vi "actionFrontEnd.vi"(6 "index":i32, 7 "editing":bool, 8 "error in (no error)":errorcluster, 9 "deviceDataBase":refnum<class "deviceDataBase.lvclass">, 10 "ScriptEventList":refnum<class "ScriptEventList.lvclass">, 11 "ActionEditor in":refnum<class "ActionEditor.lvclass">) -> (0 "error out":errorcluster, 1 "canceled":bool, 2 "ScriptEventList out":refnum<class "ScriptEventList.lvclass">, 3 "ActionEditor out":refnum<class "ActionEditor.lvclass">)   [LabVIEW 2009, in "Views.lvlib" / "ScriptEditor.lvlib" / "ActionEditor.lvclass"]
uses:
  ActionEditor.lvclass
  Tools/Scripting/ScriptingEvent/ScriptEventList/ScriptEventList.lvclass
  Tools/DatabaseHelpers/DbConnection/DeviceDataBase/deviceDataBase.lvclass
  ActionEditor.lvclass/ActionEditor.ctl
  Tools/Scripting/ScriptingEvent/ScriptEvent.lvclass
  Tools/DatabaseHelpers/Database Objects/ChannelArray/ChannelArray.lvclass
panel:
  in  "AfterEventBox":i32(listbox)
  in  "BeforeEventBox":i32[](listbox)
  in  "Stage":T1(ring)
  in  "Units":string
  in  "Delay All Events?":bool=TRUE
  in  "Comment":string
  in  "OK Button":bool
  in  "Cancel Button":bool
  in  "Channel Name":u16(ring) items=["", "Cooling_Detuning", "MOT coil", "analog2", "analog3", "analog4", "analog5", "analog6", "analog7", "analogB0", "analogB1", "analogB2", "analogB3", "analogB4", "analogB5", "analogB6", "analogB7", "Pixelfly_trigger", "Coil_Switch", "Cooling_Shutter", "Repump_Shutter", "SpinCoreDDS0_rf_trigger", "SpinCoreDDS1_rf_trigger", "CQTDDS0_rf_trigger", "Repump_AOM", "Cooling_AOM", "Imaging_Aom", "TiS", "cDDS_00", "cDDS_01", "ethernet0", "ethernet1", "ethernet2", "ethernet3"]
  in  "Action":T2(ring)
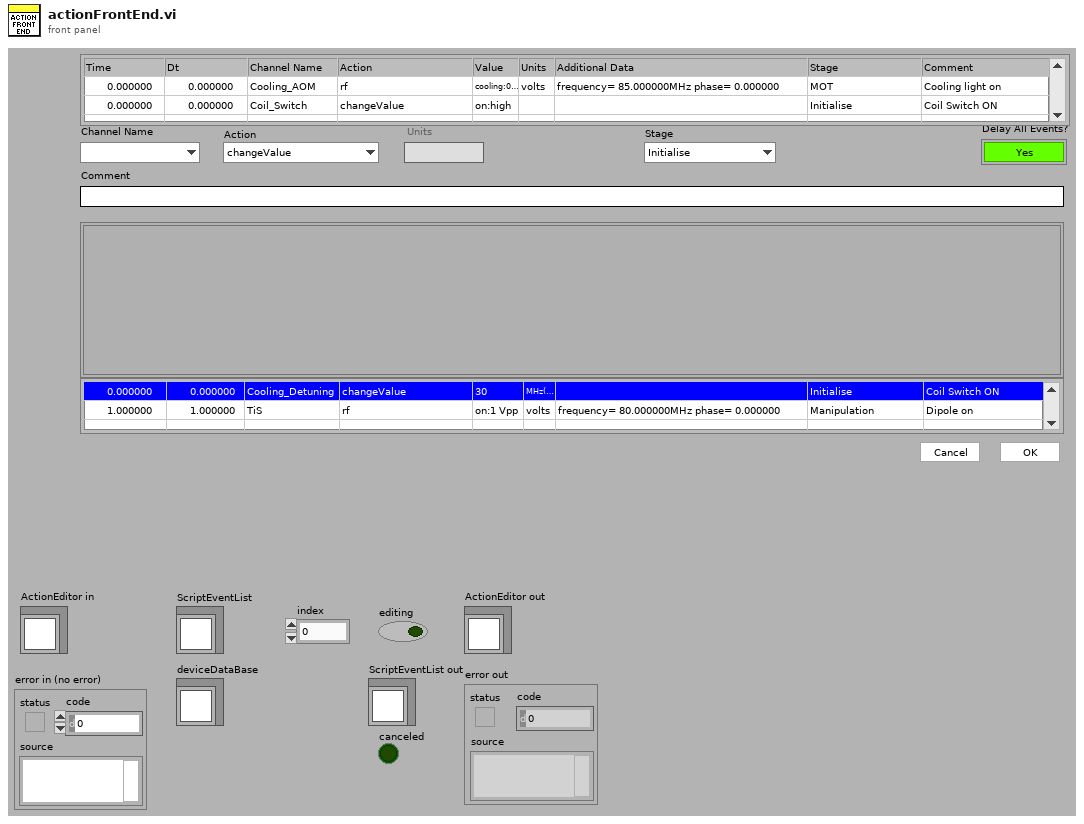
[diagram p1: front panel]
types:
  T1 = enum16{"Initialise", "MOT", "Molasses", "Optical Pumping", "Magnetic Trap", "RF Cooling", "Manipulation", "Switch Off", "Absorption Imaging", "Fluorscence Imaging", "Shut Down"}
  T2 = enum16{"changeValue", "pulse", "clock", "rampUp", "rampDown", "singleTone", "singleToneRamp", "playFile", "rf", "rfRamp"}
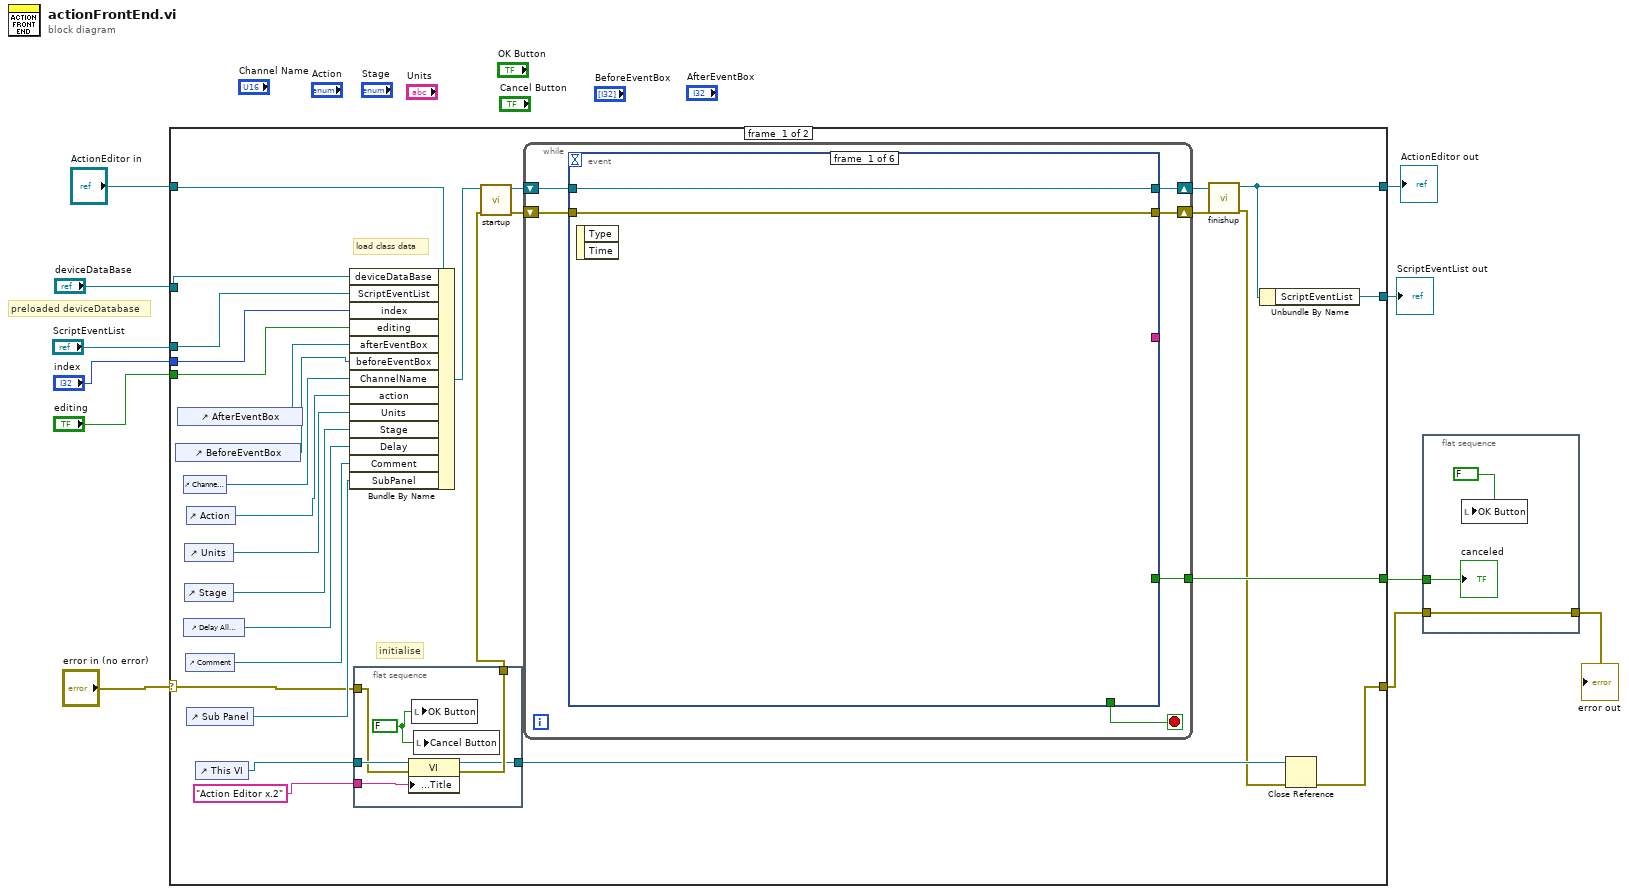
[diagram p0: block diagram]
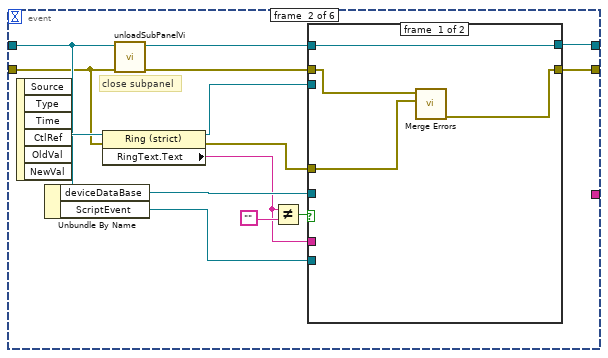
[diagram p2: hidden frame]
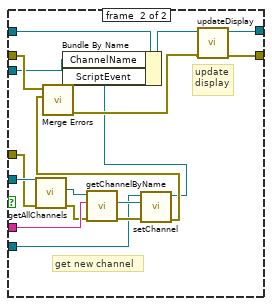
[diagram p3: hidden frame]
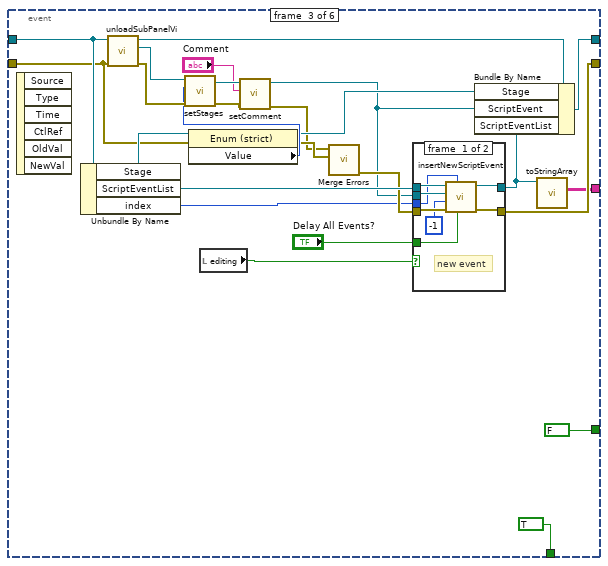
[diagram p4: hidden frame]
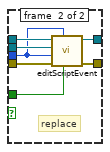
[diagram p5: hidden frame]
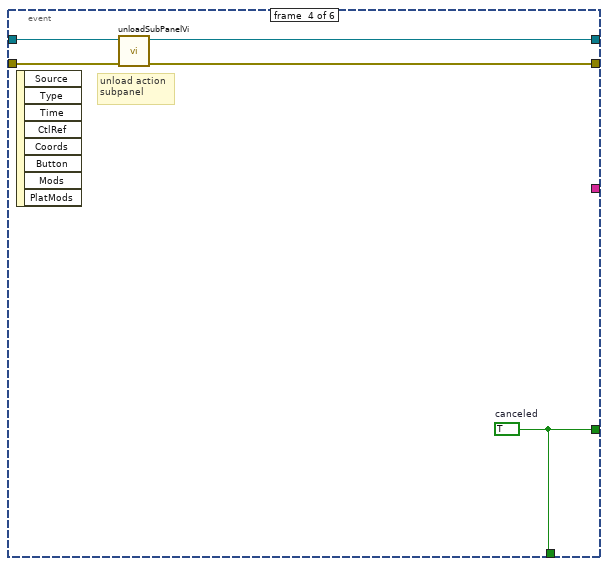
[diagram p6: hidden frame]
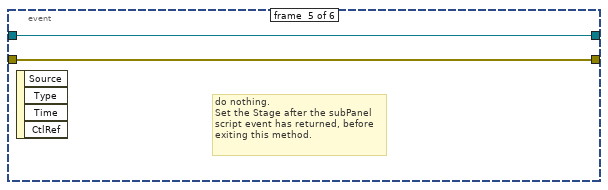
[diagram p7: hidden frame]
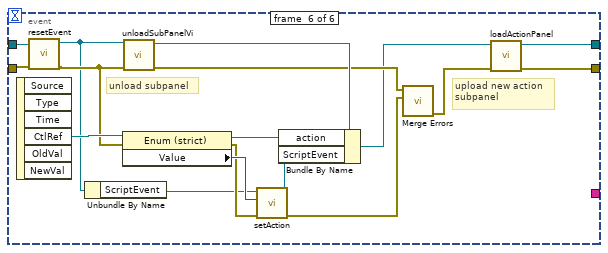
[diagram p8: hidden frame]
diagram:
  # "preloaded deviceDatabase"
  n1 = case shown="No Error" "error in (no error)" {
    selector: "error in (no error)" -> [w20 w155]
    tunnel: [w13 w155] -> w3
    tunnel: [w23 w154] -> w9
    tunnel: "ActionEditor in" -> [w36 w154]
    tunnel: "deviceDataBase" -> [w35 _]
    tunnel: "ScriptEventList" -> [w33 _]
    tunnel: "index" -> [w32 _]
    tunnel: [w24 _] -> w5
    tunnel: [w22 _] -> w4
    tunnel: "editing" -> [w18 _]
    frame #0 {
      # "initialise"
      # "load class data"
      n2 = control-ref of="BeforeEventBox"() -> (w21:refnum<vi>)
      n3 = control-ref of="AfterEventBox"() -> (w31:refnum<vi>)
      n4 = control-ref of="Channel Name"() -> (w30:refnum<vi>)
      n5 = control-ref of="Delay All Events?"() -> (w27:refnum<vi>)
      n6 = control-ref of="Units"() -> (w29:refnum<vi>)
      n7 = control-ref of="Stage"() -> (w28:refnum<vi>)
      n8 = control-ref of="Comment"() -> (w26:refnum<vi>)
      n9 = control-ref of="Action"() -> (w12:refnum<vi>)
      n10 = control-ref of="Sub Panel"() -> (w25:refnum<vi>)
      n11 = control-ref of="This VI"() -> (w17:refnum<vi>)
      n12 = Bundle By Name(cluster=w36, "deviceDataBase"=w35, "ScriptEventList"=w33, "index"=w32, "editing"=w18, "afterEventBox"=w31, "beforeEventBox"=w21, "ChannelName"=w30, "action"=w12, "Units"=w29, "Stage"=w28, "Delay"=w27, "Comment"=w26, "SubPanel"=w25) -> (w34:refnum<class "ActionEditor.lvclass">)
      n13 = flat-sequence {
        tunnel: w20 -> [w44]
        tunnel: [w43] -> w19
        tunnel: w17 -> [w45]
        tunnel: [w42] -> w15
        tunnel: "Action Editor x.2" -> [w41]
        frame #0 {
          w46 = FALSE
          n14 = property class="VI"(reference=w45, error in=w44, "Front Panel.Title"=w41) -> (reference out=w42:refnum<vi>, error out=w43:errorcluster)
          n15 = local write "OK Button"(w46) -> ()
          n16 = local write "Cancel Button"(w46) -> ()
        }
      }
      n17 = call "startup.vi"("error in (no error)"=w19, "ActionEditor in"=w34) -> ("error out"=w39:errorcluster, "ActionEditor out"=w40:refnum<class "ActionEditor.lvclass">)  [unwired: 8 in]
      n18 = while {
        shift-right: [w51] -> w37
        shift-left: w40 -> [w52]
        shift-right: [w49] -> w38
        shift-left: w39 -> [w50]
        tunnel: [w47] -> w24
        stop <- w48 stop-if-true
        n19 = event shown="[5] \"Action\": Value Change" {
          selector: _ -> [_ _ _ _ _ _]
          dyn-events: _ -> [_ _ _ _ _ _]
          timeout: _ -> [_ _ _ _ _ _]
          tunnel: [w54 w57 w100 w133 w136 w146] -> w51
          tunnel: w52 -> [w54 w67 w113 w131 w136 w140]
          tunnel: w50 -> [w53 w66 w109 w134 w135 w139]
          tunnel: [w53 w56 w102 w132 w135 w145] -> w49
          tunnel: [_ _ TRUE w130 _ _] -> w48
          tunnel: [_ _ FALSE w130 _ _] -> w47
          tunnel: [_ _ w90 _ _ _] -> _
          event #0 {
            n20 = event-data() -> ()  [unwired: 1 in, 2 out]
          }
          event #1 {
            # "close subpanel"
            n21 = event-data() -> ("CtlRef"=w68:refnum<vi>)  [unwired: 1 in, 5 out]
            n22 = Unbundle By Name(w67) -> ("deviceDataBase"=w62:refnum<class "deviceDataBase.lvclass">, "ScriptEvent"=w60:refnum<class "ScriptEvent.lvclass">)
            n23 = property class="Ring (strict)"(reference=w68, error in=w66) -> (reference out=w55:refnum<vi>, error out=w63:errorcluster, "RingText.Text"=w61:string)
            n24 = call "unloadSubPanelVi.vi"("error in (no error)"=w66, "ActionEditor in"=w67) -> ("error out"=w58:errorcluster, "ActionEditor out"=w59:refnum<class "ActionEditor.lvclass">)  [unwired: 6 in, 2 out]
            n25 = Not Equal?(x=w61, y="") -> (x != y?=w65:bool)
            n26 = case shown="True" w65 {
              tunnel: w63 -> [w70 w88]
              tunnel: w62 -> [_ w89]
              tunnel: w61 -> [_ w85]
              tunnel: w60 -> [_ w82]
              tunnel: w59 -> [w72 w79]
              tunnel: w58 -> [w71 w81]
              tunnel: [w72 w78] -> w57
              tunnel: [w69 w75] -> w56
              tunnel: w55 -> [_ w73]
              frame #0 {
                n27 = call <vilib>:"Merge Errors.vi"("error in 2 (no error)"=w70, "error in 1 (no error)"=w71) -> ("error out"=w69:errorcluster)  [unwired: 5 in]
              }
              frame #1 {
                # "update\ndisplay"
                # "get new channel"
                n28 = call "getAllChannels.vi"("error in (no error)"=w88, "deviceDataBase in"=w89) -> ("error out"=w84:errorcluster, "ChannelArray.lvclass"=w87:refnum<class "ChannelArray.lvclass">)  [unwired: 7 in, 1 out]
                n29 = call-dynamic "getChannelByName.vi"("error in (no error)"=w84, "channel_name"=w85, "ChannelArray in"=w87) -> ("error out"=w83:errorcluster, "Channel"=w86:refnum<class "Channel.lvclass">)  [unwired: 5 in, 2 out]
                n30 = call-dynamic "setChannel.vi"("error in (no error)"=w83, "Channel.lvclass"=w86, "ScriptEvent.lvclass in"=w82) -> ("error out"=w80:errorcluster, "ScriptEvent.lvclass out"=w74:refnum<class "ScriptEvent.lvclass">)  [unwired: 7 in]
                n31 = call <vilib>:"Merge Errors.vi"("error in 2 (no error)"=w80, "error in 1 (no error)"=w81) -> ("error out"=w76:errorcluster)  [unwired: 5 in]
                n32 = Bundle By Name(cluster=w79, "ChannelName"=w73, "ScriptEvent"=w74) -> (w77:refnum<class "ActionEditor.lvclass">)
                n33 = call "updateDisplay.vi"("error in (no error)"=w76, "ActionEditor in"=w77) -> ("error out"=w75:errorcluster, "ActionEditor out"=w78:refnum<class "ActionEditor.lvclass">)  [unwired: 8 in]
              }
            }
          }
          event #2 {
            n34 = event-data() -> ()  [unwired: 1 in, 6 out]
            n35 = Unbundle By Name(w113) -> ("Stage"=w110:refnum<vi>, "ScriptEventList"=w106:refnum<class "ScriptEventList.lvclass">, "index"=w104:i32)
            n36 = call "unloadSubPanelVi.vi"("error in (no error)"=w109, "ActionEditor in"=w113) -> ("error out"=w111:errorcluster, "ScriptEvent"=w112:refnum<class "ScriptEvent.lvclass">, "ActionEditor out"=w101:refnum<class "ActionEditor.lvclass">)  [unwired: 6 in, 1 out]
            n37 = property class="Enum (strict)"(reference=w110, error in=w109) -> (reference out=w103:refnum<vi>, error out=w107:errorcluster, "Value"=w108:T1)
            n38 = call-dynamic "setStages.vi"("error in (no error)"=w111, "Stage"=w108, "ScriptEvent.lvclass in"=w112) -> ("error out"=w97:errorcluster, "ScriptEvent.lvclass out"=w98:refnum<class "ScriptEvent.lvclass">)  [unwired: 7 in]
            n39 = local read "editing"() -> (w92:bool)
            n40 = call-dynamic "setComment.vi"("error in (no error)"=w97, "comment"="Comment", "ScriptEvent.lvclass in"=w98) -> ("error out"=w96:errorcluster, "ScriptEvent.lvclass out"=w95:refnum<class "ScriptEvent.lvclass">)  [unwired: 7 in]
            n41 = call <vilib>:"Merge Errors.vi"("error in 2 (no error)"=w107, "error in 1 (no error)"=w96) -> ("error out"=w105:errorcluster)  [unwired: 5 in]
            n42 = case shown="True" w92 {
              tunnel: w106 -> [w122 w127]
              tunnel: w105 -> [w118 w125]
              tunnel: w104 -> [w116 w123]
              tunnel: [w121 w129] -> w91
              tunnel: [w120 w128] -> w102
              tunnel: w95 -> [w119 w126]
              tunnel: "Delay All Events?" -> [w117 w124]
              frame #0 {
                # "new event"
                n43 = call "insertNewScriptEvent.vi"("delayAll"=w117, "selectedIndex"=w116, "error in (no error)"=w118, "index"=-1, "ScriptEvent"=w119, "ScriptEventList in"=w122) -> ("error out"=w120:errorcluster, "ScriptEventList out"=w121:refnum<class "ScriptEventList.lvclass">)  [unwired: 4 in]
              }
              frame #1 {
                # "replace"
                n44 = call "editScriptEvent.vi"("delayAll"=w124, "selectedIndex"=w123, "error in (no error)"=w125, "index"=w123, "ScriptEvent"=w126, "ScriptEventList in"=w127) -> ("error out"=w128:errorcluster, "ScriptEventList out"=w129:refnum<class "ScriptEventList.lvclass">)  [unwired: 4 in]
              }
            }
            n45 = Bundle By Name(cluster=w101, "Stage"=w103, "ScriptEvent"=w95, "ScriptEventList"=w91) -> (w100:refnum<class "ActionEditor.lvclass">)
            n46 = call "toStringArray.vi"("ScriptEventList in"=w91) -> ("Array"=w90:string[][])  [unwired: 8 in, 2 out]
          }
          event #3 {
            w130 = TRUE  # canceled
            # "unload action\nsubpanel"
            n47 = event-data() -> ()  [unwired: 1 in, 8 out]
            n48 = call "unloadSubPanelVi.vi"("error in (no error)"=w134, "ActionEditor in"=w131) -> ("error out"=w132:errorcluster, "ActionEditor out"=w133:refnum<class "ActionEditor.lvclass">)  [unwired: 6 in, 2 out]
          }
          event #4 {
            # "do nothing.\nSet the Stage after the subPanel\nscript event has returned, before\nexiting this method."
            n49 = event-data() -> ()  [unwired: 1 in, 4 out]
          }
          event #5 {
            # "upload new action\nsubpanel"
            # "unload subpanel"
            n50 = event-data() -> ("CtlRef"=w152:refnum<vi>)  [unwired: 1 in, 5 out]
            n51 = call "resetEvent.vi"("error in (no error)"=w139, "ActionEditor in"=w140) -> ("error out"=w141:errorcluster, "ActionEditor out"=w138:refnum<class "ActionEditor.lvclass">)  [unwired: 8 in]
            n52 = Unbundle By Name(w138) -> ("ScriptEvent"=w144:refnum<class "ScriptEvent.lvclass">)
            n53 = property class="Enum (strict)"(reference=w152, error in=w141) -> (reference out=w137:refnum<vi>, error out=w150:errorcluster, "Value"=w151:T2)
            n54 = call "unloadSubPanelVi.vi"("error in (no error)"=w141, "ActionEditor in"=w138) -> ("error out"=w148:errorcluster, "ActionEditor out"=w153:refnum<class "ActionEditor.lvclass">)  [unwired: 6 in, 2 out]
            n55 = call "setAction.vi"("error in (no error)"=w150, "action"=w151, "ScriptEvent.lvclass in"=w144) -> ("error out"=w147:errorcluster, "ScriptEvent.lvclass out"=w149:refnum<class "ScriptEvent.lvclass">)  [unwired: 7 in]
            n56 = Bundle By Name(cluster=w153, "action"=w137, "ScriptEvent"=w149) -> (w143:refnum<class "ActionEditor.lvclass">)
            n57 = call <vilib>:"Merge Errors.vi"("error in 2 (no error)"=w147, "error in 1 (no error)"=w148) -> ("error out"=w142:errorcluster)  [unwired: 5 in]
            n58 = call "loadActionPanel.vi"("error in (no error)"=w142, "ActionEditor in"=w143) -> ("error out"=w145:errorcluster, "ActionEditor out"=w146:refnum<class "ActionEditor.lvclass">)  [unwired: 8 in]
          }
        }
      }
      n59 = call "finishup.vi"("error in (no error)"=w38, "ActionEditor in"=w37) -> ("error out"=w14:errorcluster, "ActionEditor out"=w23:refnum<class "ActionEditor.lvclass">)  [unwired: 8 in]
      n60 = Unbundle By Name(w23) -> ("ScriptEventList"=w22:refnum<class "ScriptEventList.lvclass">)
      n61 = Close Reference(reference=w15, error in (no error)=w14) -> (error out=w13:errorcluster)
    }
    frame #1 {
    }
  }
  "ActionEditor out" <- w9
  "ScriptEventList out" <- w4
  n62 = flat-sequence {
    tunnel: w5 -> [w158]
    tunnel: w3 -> [w156]
    tunnel: [w156] -> w2
    frame #0 {
      n63 = local write "OK Button"(FALSE) -> ()
      "canceled" <- w158
    }
  }
  "error out" <- w2
